vi "New Report.vi"(8 "error in":errorcluster, 11 "Report Generator in":refnum<class "Report Generator.lvclass">) -> (0 "error out":errorcluster, 3 "Report Generator out":refnum<class "Report Generator.lvclass">)   [LabVIEW 2023, in "Report Generator.lvlib" / "Report Generator.lvclass"]
uses:
  Library/Report Generator.lvclass
  C:/Users/Public/Documents/Development/builds/Engine/Engine.lvlibp/Project/Engine.lvclass
  builds/Engine/Engine.lvlibp/Accessors/Read Report Queue.vi
  builds/Tools/QDMH.lvlibp/QDMH.lvclass
  builds/Engine/Engine.lvlibp/Project/Engine.lvclass
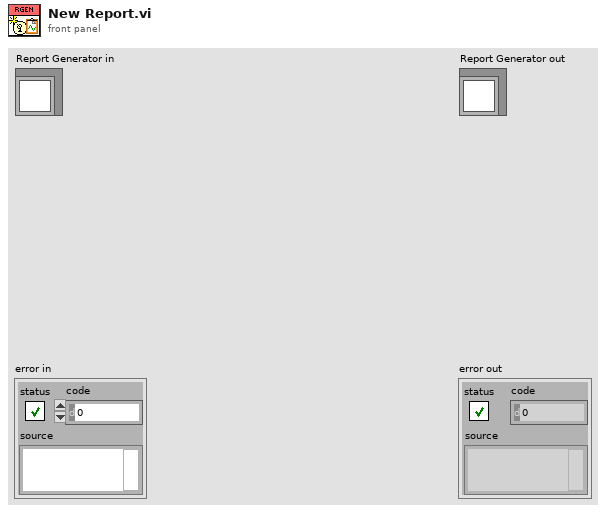
[diagram p1: front panel]
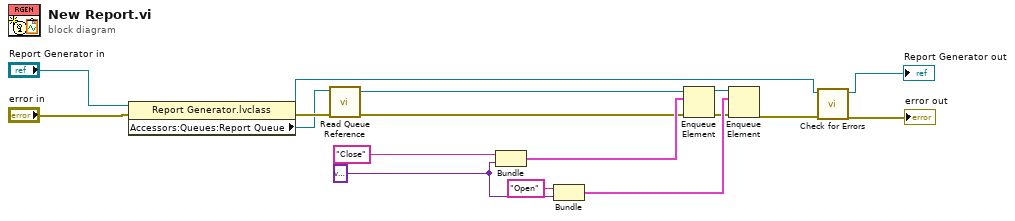
[diagram p0: block diagram]
diagram:
  w14 = variant
  n1 = property class="Report Generator.lvclass"(reference="Report Generator in", error in="error in") -> (reference out=w17:refnum<class "Report Generator.lvclass">, error out=w8:errorcluster, "Accessors:Queues:Report Queue"=w6:refnum<class "QDMH.lvclass">)
  n2 = call "Read Queue Reference.vi"("error in"=w8, "QDMH in"=w6) -> ("error out"=w9:errorcluster, "Queue Reference"=w7:refnum<queue>)  [unwired: 7 in, 1 out]
  n3 = Bundle("Close", w14) -> (w10:cluster{string, variant})  [unwired: 1 in]
  n4 = Bundle("Open", w14) -> (w13:cluster{string, variant})  [unwired: 1 in]
  n5 = Enqueue Element(queue=w7, element=w10, error in (no error)=w9) -> (queue out=w12:refnum<queue>, error out=w11:errorcluster)  [unwired: 1 in, 1 out]
  n6 = Enqueue Element(queue=w12, element=w13, error in (no error)=w11) -> (error out=w16:errorcluster)  [unwired: 1 in, 2 out]
  n7 = call "Check for Errors.vi"("error in"=w16, "Engine in"=w17) -> ("error out"=→"error out":errorcluster, "Engine out"=→"Report Generator out":refnum<class "Report Generator.lvclass">)  [unwired: 8 in]
